vi "init_ROI.vi"(2 "Input ROI Array":dbl[][](array[numeric]), 3 "camera cluster":T3) -> (0 "First Call? out":bool, 1 "Output ROI Array":dbl[][](array[numeric]))   [LabVIEW 2015]
uses:
  <vilib>/vision/Avi1.llb/AviRefnum.ctl
  <vilib>/userdefined/High Color/IMAQdx.ctl
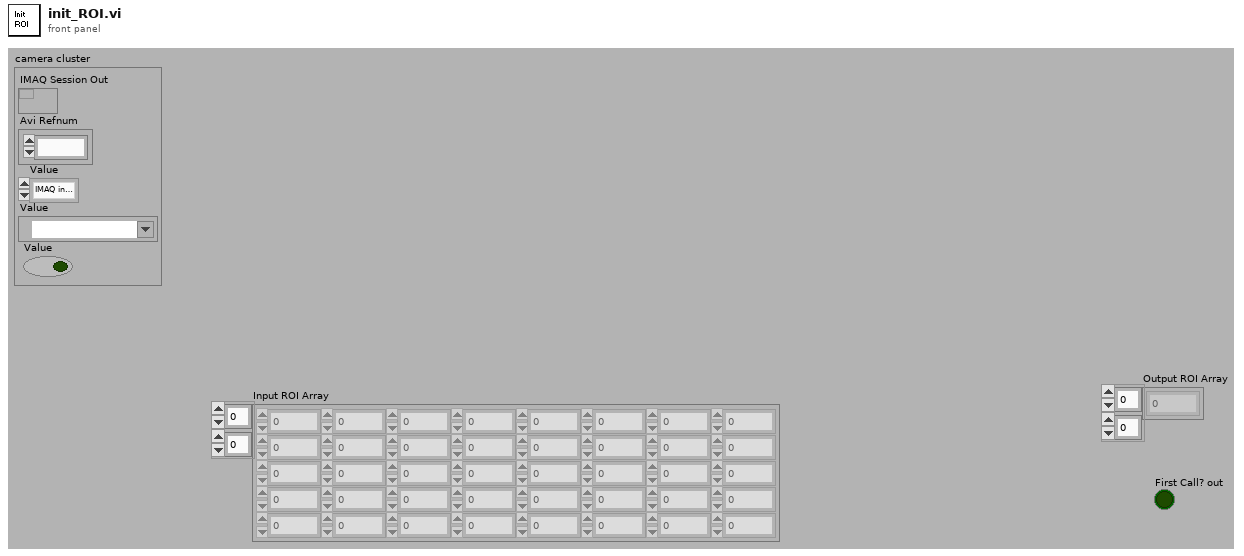
[diagram p1: front panel]
types:
  T1 = typedef "AviRefnum.ctl" = refnum<k1>
  T2 = typedef "IMAQdx.ctl" = refnum<k21>
  T3 = cluster{"IMAQ Session Out":refnum<k11>, "Avi Refnum":T1, "Value":enum32{"IMAQ interface", "IMAQdx interface", "AVI file"}, "Value":T2, "Value":bool}
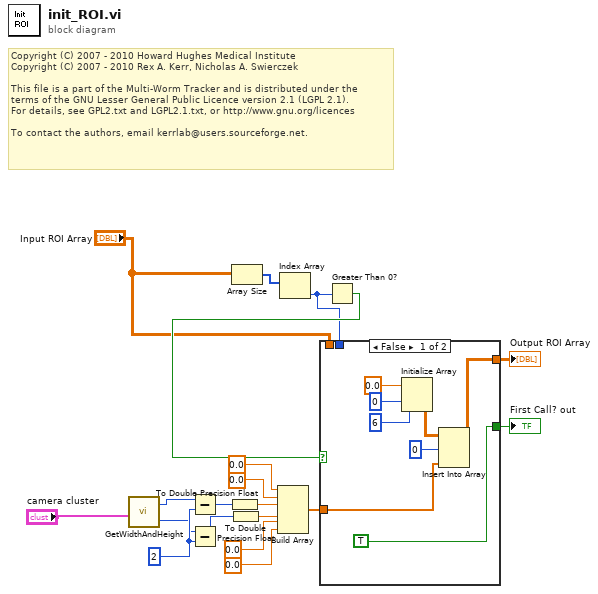
[diagram p0: block diagram]
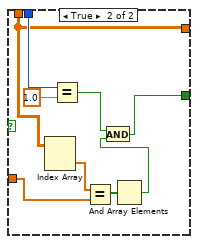
[diagram p2: hidden frame]
diagram:
  w4 = u32 2 ("y")
  # "Copyright (C) 2007 - 2010 Howard Hughes Medical Institute\nCopyright (C) 2007 - 2010 Rex A. Kerr, Nicholas A. Swierczek\n \nThis file is a part of the Multi-Worm Tracker and is distributed under the\nterms of the GNU Lesser General Public Licence version 2.1 (LGPL 2.1).\nFor details, see GPL2.txt and LGPL2.1.txt, or http://www.gnu.org/licences\n \nTo contact the authors, email kerrlab@users.sourceforge.net."
  n1 = call "GetWidthAndHeight.vi"("camera cluster"="camera cluster") -> ("Width"=w3:u32, "Height"=w2:u32)
  n2 = Subtract(x=w3, y=w4) -> (x-y=w13:u32)
  n3 = Subtract(x=w2, y=w4) -> (x-y=w14:u32)
  n4 = To Double Precision Float(number=w13) -> (double precision float=w11:dbl)
  n5 = To Double Precision Float(number=w14) -> (double precision float=w12:dbl)
  n6 = Array Size(array="Input ROI Array") -> (size(s)=w19:i32[])
  n7 = Build Array(0.0, 0.0, w11, w12, 0.0, 0.0) -> (w8:dbl[])
  n8 = Index Array(array=w19) -> (element=w17:i32)  [unwired: 1 in]
  n9 = Greater Than 0?(x=w17) -> (x > 0?=w18:bool)
  n10 = case shown="False" w18 {
    tunnel: [w22 w34] -> w6
    tunnel: "Input ROI Array" -> [_ w34]
    tunnel: w17 -> [_ w35]
    tunnel: w8 -> [w21 w32]
    tunnel: [TRUE w28] -> w5
    frame False {
      n11 = Initialize Array(0.0 ("element"), 0 ("dimension size"), 6 ("dimension size")) -> (w24:dbl[][])
      n12 = Insert Into Array(array=w24, index (row)=0, new element=w21) -> (w22:dbl[][])  [unwired: 1 in]
    }
    frame True {
      n13 = Index Array(array=w34) -> (element=w33:dbl[])  [unwired: 2 in]
      n14 = Equal?(x=w35, y=1.0) -> (x = y?=w29:bool)
      n15 = Equal?(x=w33, y=w32) -> (x = y?=w31:bool[])
      n16 = And Array Elements(Boolean array=w31) -> (logical AND=w30:bool)
      n17 = And(x=w29, y=w30) -> (x .and. y?=w28:bool)
    }
  }
  "Output ROI Array" <- w6
  "First Call? out" <- w5
